vi "Full LabView Code.vi"() -> ()   [LabVIEW 2020]
uses:
  C:/Program Files (x86)/National Instruments/LabVIEW 2020/examples/Connectivity/Python/support/PythonVersionsEnum.ctl
  <vilib>/Utility/miscctls.llb/LVRectTypeDef.ctl
  <vilib>/Utility/miscctls.llb/LVPointTypeDef.ctl
  <vilib>/Instr/_visa.llb/VISA Configure Serial Port (Instr).vi
panel:
  out "final_calc":dbl
  out "Python error out":errorcluster
  in  "Python version":T1=enum."3.6"
  out "Suggested Min Electrode Separation (mm)":dbl format="%#_2g"
  out "Time for Evaporation":dbl
  out "Evaporation Rate":dbl
  out "droplet size":dbl
  out "Initial Droplet Charge":dbl
  out "Current":dbl
  in  "Flow Rate (L/min)":dbl=5e-05 min=0.0 max=1.0 step=1e-06
  in  "Voltage (V)":dbl=5000.0 min=0.0 max=5000.0 step=10.0
  in  "Solvent":enum16{"Xylene"}(ring)
  in  "Electrode separation (mm)":dbl(slide)=5.0 min=1.0 max=65.0 step=1.0
  out "Arduino Error Out":errorcluster
  out "Arduino Serial Return":string
  in  "Set":bool
  in  "Arduino COM Port":refnum<visa-resource-name>="COM5"
  in  "Stop":bool
  # "Setup"
  # "Stage Control"
  # "Spray Modelling"
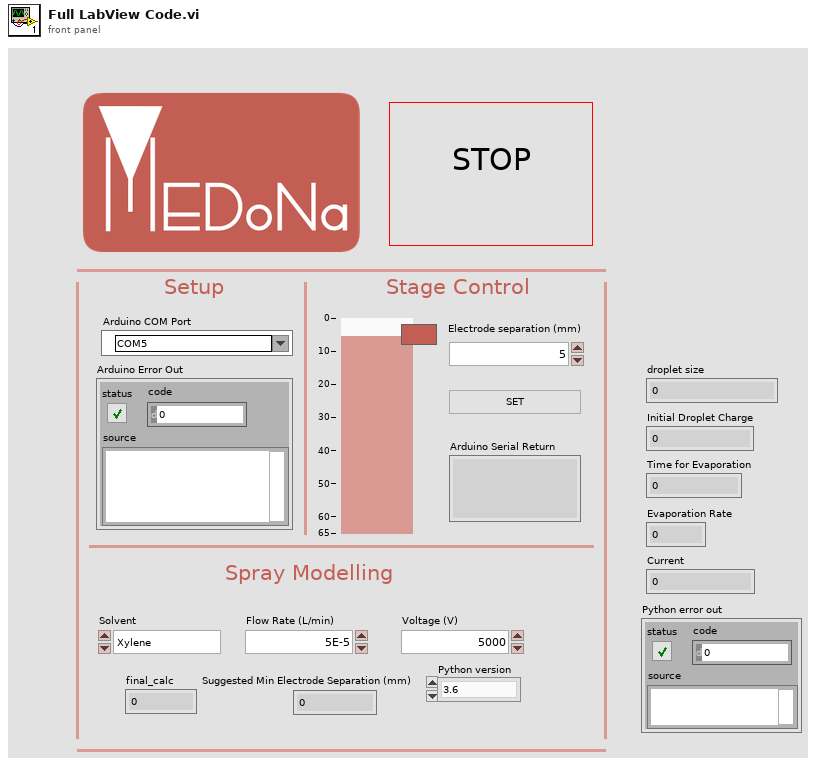
[diagram p1: front panel]
types:
  T1 = typedef "PythonVersionsEnum.ctl" = enum16{"2.7", "3.6"}
  T2 = typedef "LVRectTypeDef.ctl" = cluster{"Left":i16, "Top":i16, "Right":i16, "Bottom":i16}
  T3 = typedef "LVPointTypeDef.ctl" = cluster{"Horizontal":i16, "Vertical":i16}
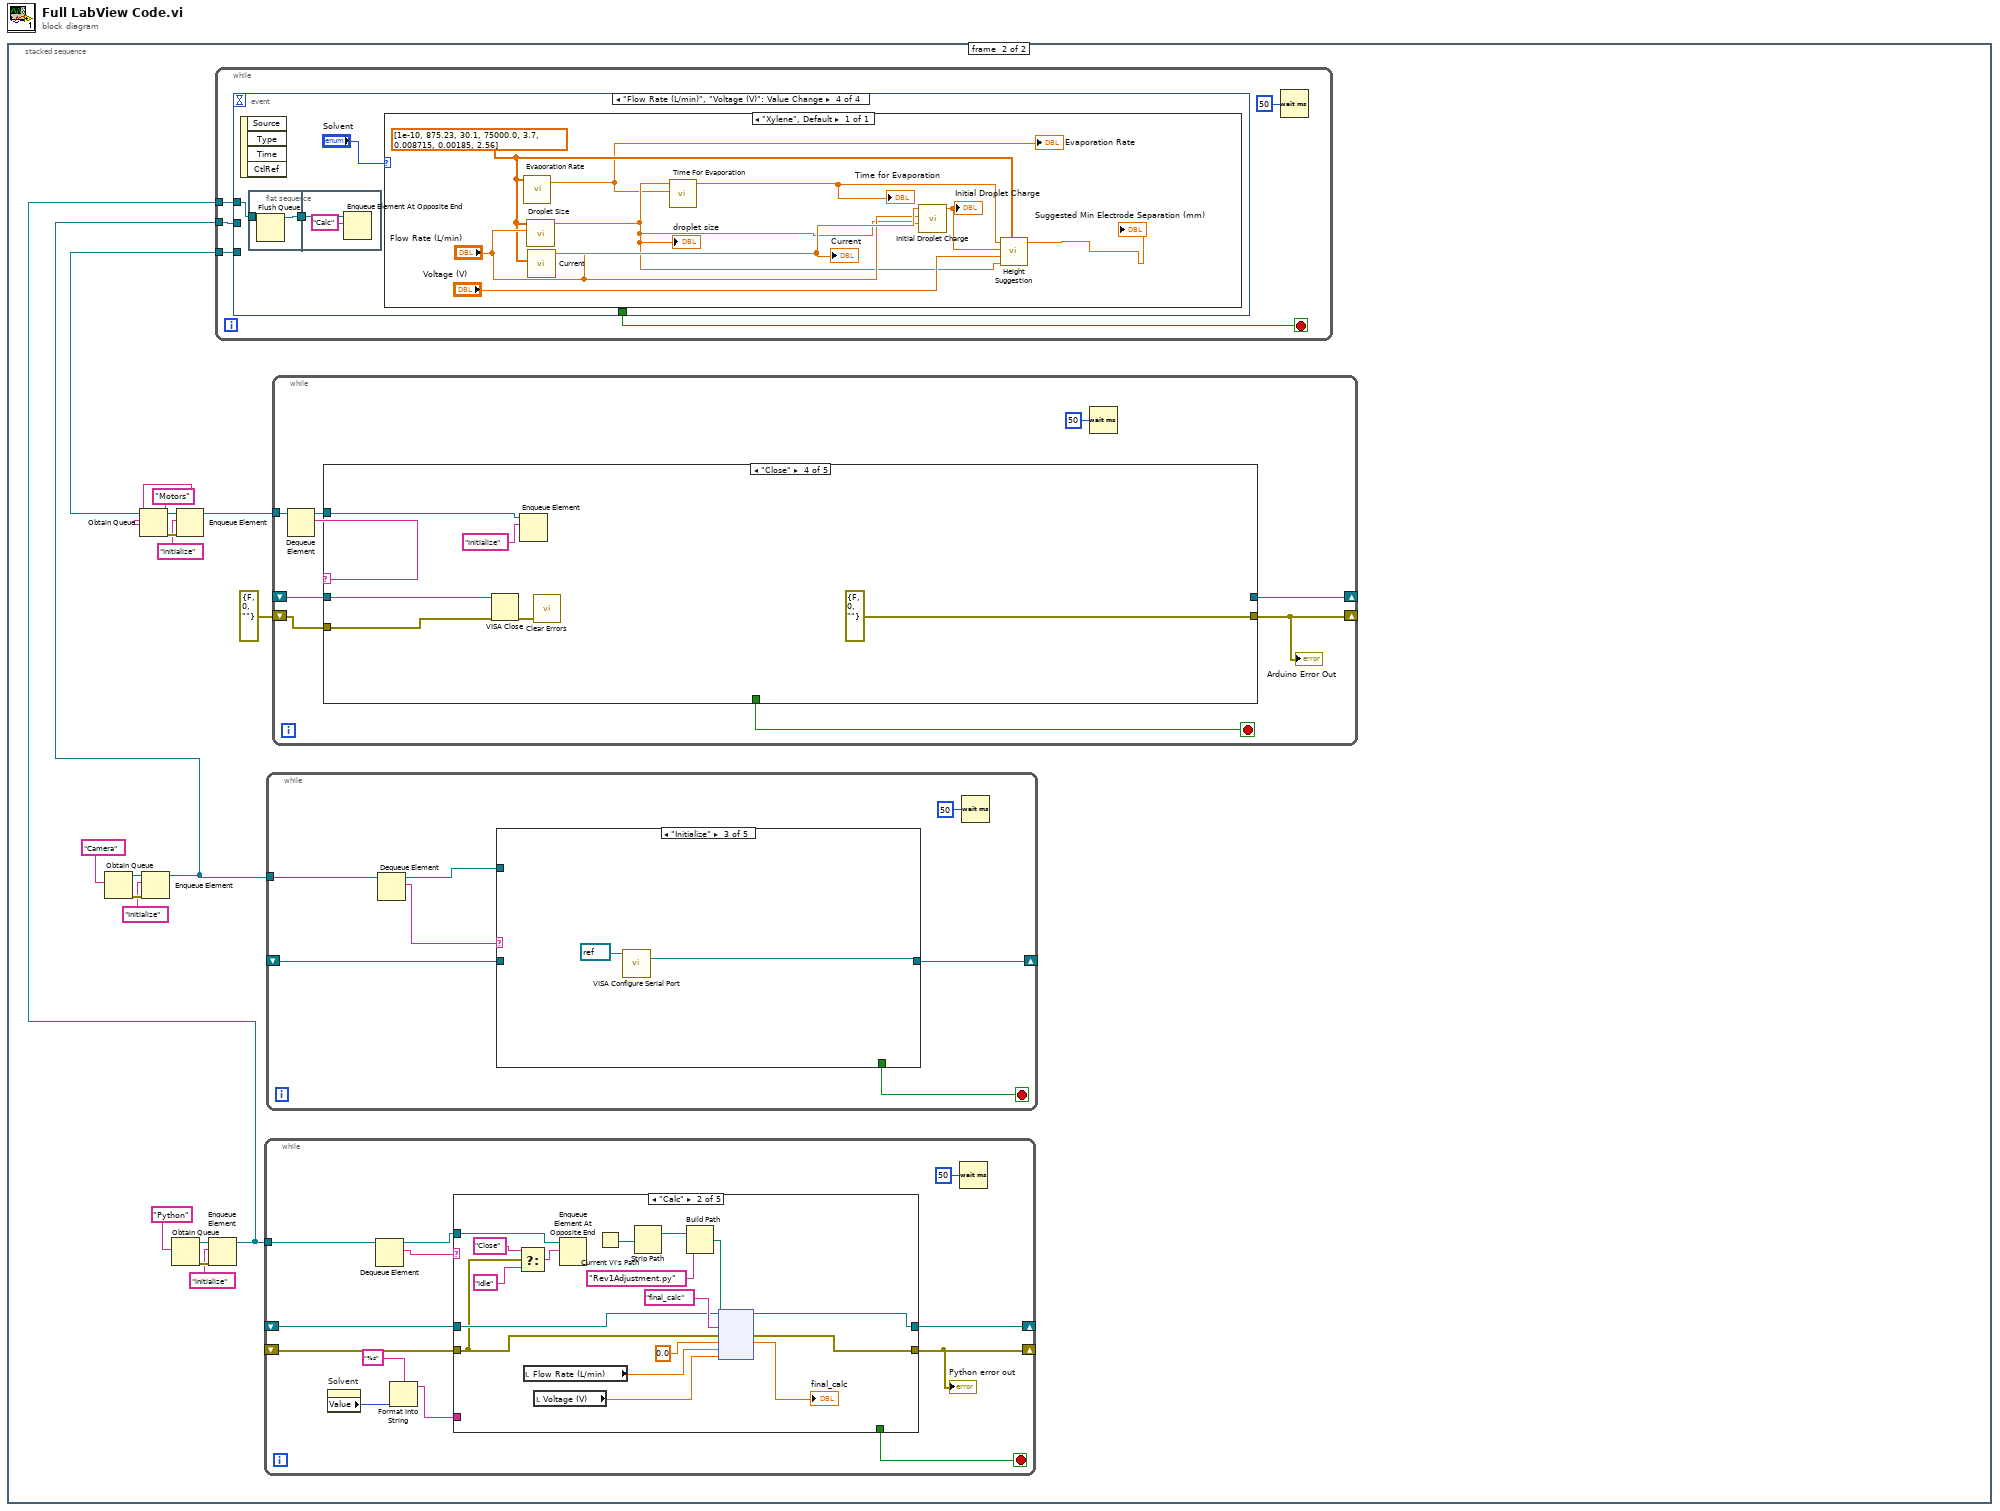
[diagram p0: block diagram]
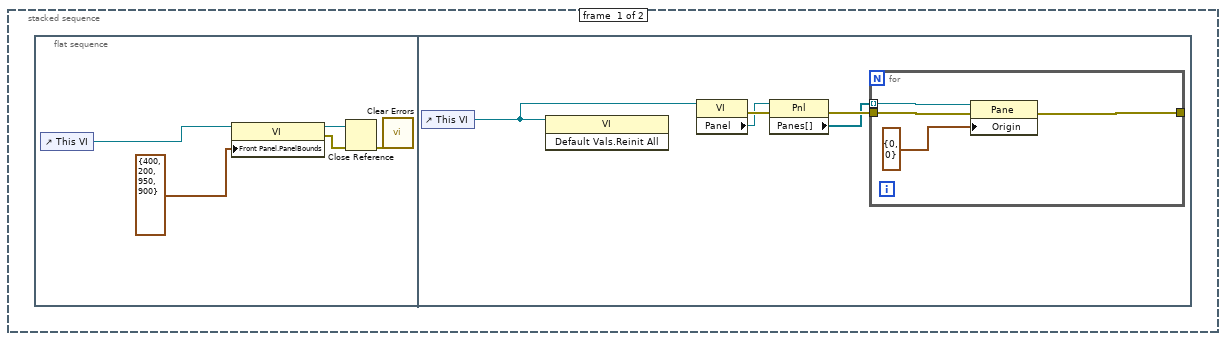
[diagram p2: hidden frame]
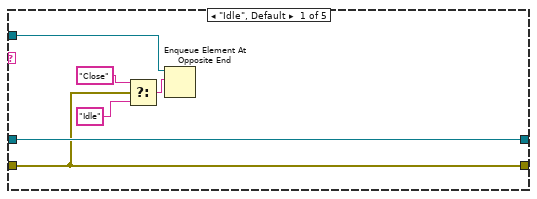
[diagram p3: hidden frame]
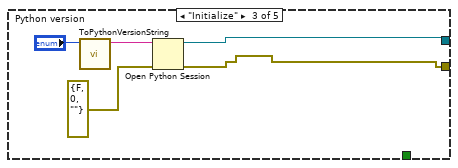
[diagram p4: hidden frame]
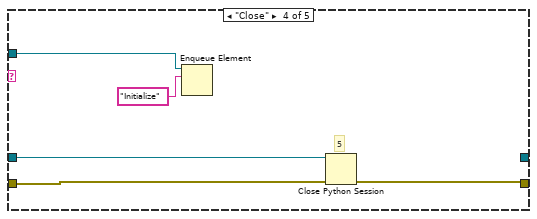
[diagram p5: hidden frame]
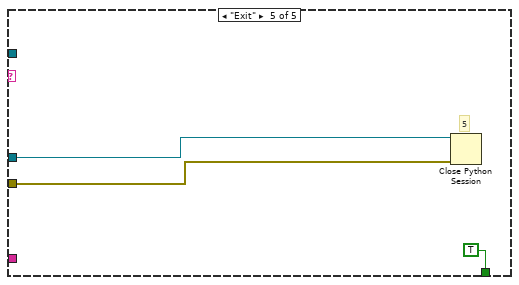
[diagram p6: hidden frame]
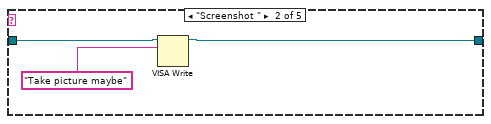
[diagram p8: hidden frame]
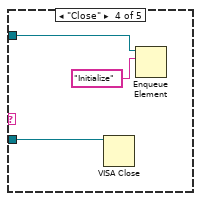
[diagram p9: hidden frame]
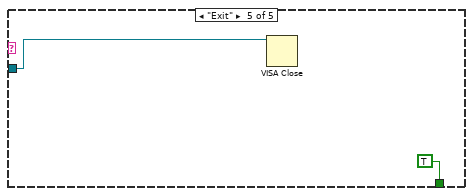
[diagram p10: hidden frame]
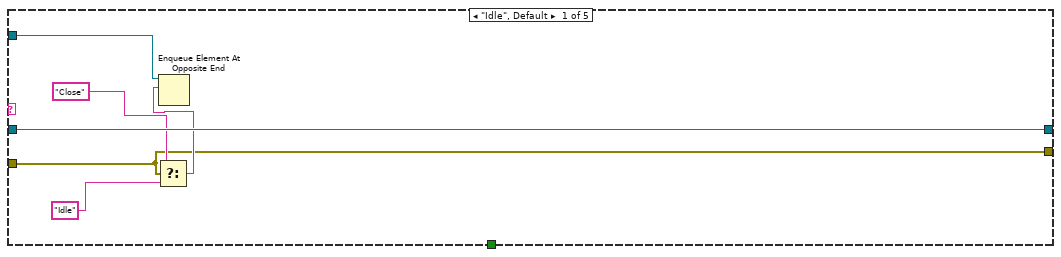
[diagram p11: hidden frame]
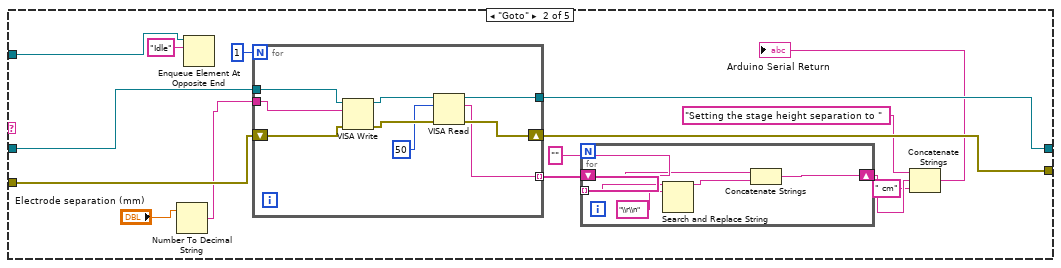
[diagram p12: hidden frame]
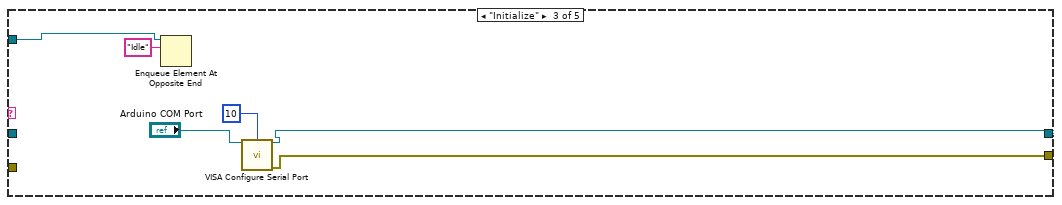
[diagram p13: hidden frame]
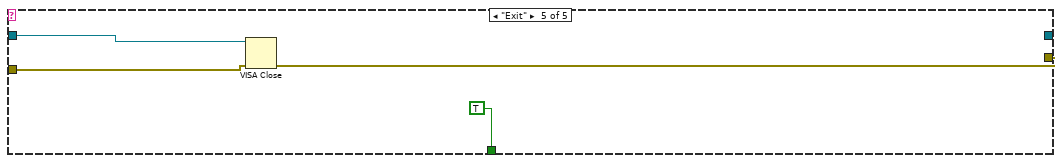
[diagram p14: hidden frame]
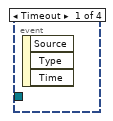
[diagram p15: hidden frame]
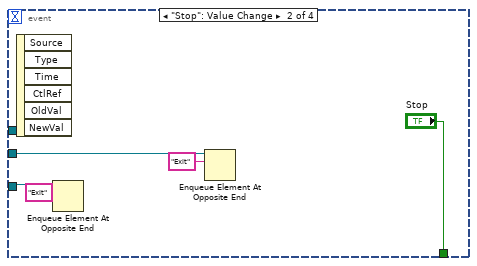
[diagram p16: hidden frame]
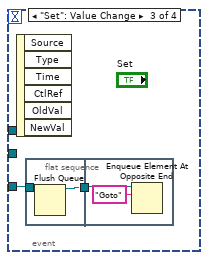
[diagram p17: hidden frame]
diagram:
  n1 = stacked-sequence {
    frame #0 {
      n2 = flat-sequence {
        frame #0 {
          n3 = control-ref of="This VI"() -> (w3:refnum<vi>)
          n4 = property class="VI"(reference=w3, "Front Panel.PanelBounds"=T2 {"Left"=400, "Top"=200, "Right"=950, "Bottom"=900} ("Front Panel Window:Panel Bounds")) -> (reference out=w5:refnum<vi>, error out=w4:errorcluster)  [unwired: 1 in]
          n5 = Close Reference(reference=w5, error in (no error)=w4) -> (error out=w1:errorcluster)
          n6 = call <vilib>:"Clear Errors.vi"("error in (no error)"=w1) -> ()  [unwired: 5 in, 2 out]
        }
        frame #1 {
          n7 = control-ref of="This VI"() -> (w10:refnum<vi>)
          n8 = invoke class="VI" method="Default Vals.Reinit All"(reference=w10) -> ()  [unwired: 2 in, 3 out]
          n9 = property class="VI"(reference=w10) -> (error out=w7:errorcluster, "Panel"=w6:refnum<vi>)  [unwired: 1 in, 1 out]
          n10 = property class="Pnl"(reference=w6, error in=w7) -> (error out=w9:errorcluster, "Panes[]"=w8:refnum<vi>[])  [unwired: 1 out]
          n11 = for {
            tunnel: w8 -> [w14] mode=indexing
            tunnel: w9 -> [w13]
            tunnel: [w11] -> _
            n12 = property class="Pane"(reference=w14, error in=w13, "Origin"=T3 {"Horizontal"=0, "Vertical"=0}) -> (error out=w11:errorcluster)  [unwired: 1 out]
          }
        }
      }
    }
    frame #1 {
      w28 = "Motors" ("name (unnamed)")
      n13 = Obtain Queue(element data type="Camera" ("name (unnamed)")) -> (queue out=w22:refnum<queue>, error out=w25:errorcluster)  [unwired: 4 in, 1 out]
      n14 = Obtain Queue(name (unnamed)=w28, element data type=w28) -> (queue out=w27:refnum<queue>, error out=w30:errorcluster)  [unwired: 3 in, 1 out]
      n15 = Enqueue Element(queue=w22, element="Initialize", error in (no error)=w25) -> (queue out=w21:refnum<queue>)  [unwired: 1 in, 2 out]
      n16 = Obtain Queue(element data type="Python" ("name (unnamed)")) -> (queue out=w16:refnum<queue>, error out=w19:errorcluster)  [unwired: 4 in, 1 out]
      n17 = Enqueue Element(queue=w27, element="Initialize", error in (no error)=w30) -> (queue out=w26:refnum<queue>)  [unwired: 1 in, 2 out]
      n18 = Enqueue Element(queue=w16, element="Initialize", error in (no error)=w19) -> (queue out=w15:refnum<queue>)  [unwired: 1 in, 2 out]
      n19 = while {
        tunnel: w27 -> [w161]
        tunnel: w21 -> [w160]
        tunnel: w15 -> [w157]
        stop <- w159 stop-if-true
        n20 = event shown="[3] \"Flow Rate (L/min)\", \"Voltage (V)\": Value Change" {
          selector: _ -> [_ _ _ _]
          dyn-events: _ -> [_ _ _ _]
          timeout: _ -> [_ _ _ _]
          tunnel: w161 -> [_ w164 w168 _]
          tunnel: w160 -> [_ w165 _ _]
          tunnel: [_ "Stop" _ _] -> w159
          tunnel: w157 -> [_ _ _ w173]
          event Timeout {
            n21 = event-data() -> ()  [unwired: 1 in, 3 out]
          }
          event "Stop": Value Change {
            n22 = event-data() -> ()  [unwired: 1 in, 6 out]
            n23 = Enqueue Element At Opposite End(queue=w164, element="Exit") -> ()  [unwired: 2 in, 3 out]
            n24 = Enqueue Element At Opposite End(queue=w165, element="Exit") -> ()  [unwired: 2 in, 3 out]
          }
          event "Set": Value Change {
            n25 = event-data() -> ()  [unwired: 1 in, 6 out]
            n26 = flat-sequence {
              tunnel: w168 -> [w170]
              tunnel: [w169] -> w167
              tunnel: w167 -> [w171]
              frame #0 {
                n27 = Flush Queue(queue=w170) -> (queue out=w169:refnum<queue>)  [unwired: 1 in, 2 out]
              }
              frame #1 {
                n28 = Enqueue Element At Opposite End(queue=w171, element="Goto") -> ()  [unwired: 2 in, 3 out]
              }
            }
          }
          event "Flow Rate (L/min)", "Voltage (V)": Value Change {
            n29 = event-data() -> ()  [unwired: 1 in, 4 out]
            n30 = flat-sequence {
              tunnel: w173 -> [w177]
              tunnel: [w176] -> w174
              tunnel: w174 -> [w178]
              frame #0 {
                n31 = Flush Queue(queue=w177) -> (queue out=w176:refnum<queue>)  [unwired: 1 in, 2 out]
              }
              frame #1 {
                n32 = Enqueue Element At Opposite End(queue=w178, element="Calc") -> ()  [unwired: 2 in, 3 out]
              }
            }
            n33 = case shown="\"Xylene\", Default" "Solvent" {
              frame "Xylene", Default {
                w182 = dbl[] [1e-10, 875.23, 30.1, 75000.0, 3.7, 0.008715, 0.00185, 2.56] ("Array 2")
                n34 = call "Evaporation Rate.vi"("array"=w182) -> ("Evaporation Rate"=w181:dbl)  [unwired: 10 in]
                "Evaporation Rate" <- w181
                n35 = call "Droplet Size.vi"("Flow Rate"="Flow Rate (L/min)", "Array"=w182) -> ("droplet size"=w183:dbl)  [unwired: 9 in]
                "droplet size" <- w183
                n36 = call "Current.vi"("array"=w182, "Flow Rate (uL/min)"="Flow Rate (L/min)") -> ("Current"=w188:dbl)  [unwired: 9 in]
                "Current" <- w188
                n37 = call "Time For Evaporation.vi"("Evaporation rate"=w181, "Droplet Size"=w183) -> ("Time for Evaporation"=w186:dbl)  [unwired: 9 in]
                "Time for Evaporation" <- w186
                n38 = call "Initial Droplet Charge.vi"("Droplet Size"=w183, "Flow Rate"="Flow Rate (L/min)", "Current"=w188) -> ("Initial Droplet Charge"=w185:dbl)  [unwired: 8 in]
                "Initial Droplet Charge" <- w185
                n39 = call "Height Suggestion.vi"("array"=w182, "Droplet Size"=w183, "Input Voltage"="Voltage (V)", "Initial Charge"=w185, "Evaporation Time"=w186) -> ("Suggested Height"=→"Suggested Min Electrode Separation (mm)":dbl)  [unwired: 6 in]
              }
            }
          }
        }
        n40 = Wait (ms)(milliseconds to wait=u32 50) -> ()  [unwired: 1 out]
      }
      n41 = while {
        tunnel: w15 -> [w42]
        shift-right: [w37] -> _
        shift-left: _ -> [w35]
        shift-right: [w34] -> _
        shift-left: _ -> [w36]
        stop <- w39 stop-if-true
        n42 = property on="Solvent" class="Enum (strict)"() -> ("Value"=w33:enum16{"Xylene"})  [unwired: 2 in, 2 out]
        n43 = Dequeue Element(queue=w42) -> (queue out=w41:refnum<queue>, element=w40:string)  [unwired: 2 in, 2 out]
        n44 = Format Into String(format string="%s", w33) -> (resulting string=w31:string)  [unwired: 2 in, 1 out]
        n45 = case shown="\"Calc\"" w40 {
          tunnel: w41 -> [w45 w49 _ w75 _]
          tunnel: [_ _ _ _ TRUE] -> w39
          tunnel: [w44 w58 w67 _ _] -> w37
          tunnel: [w43 w59 w66 w71 _] -> w34
          tunnel: w36 -> [w43 w50 _ w73 w76]
          tunnel: w35 -> [w44 w60 _ w72 w77]
          tunnel: w31 -> [_ _ _ _ _]
          frame "Idle", Default {
            n46 = Select(t="Close", s=w43, f="Idle" ("element")) -> (s? t:f=w46:string)
            n47 = Enqueue Element At Opposite End(queue=w45, element=w46) -> ()  [unwired: 2 in, 3 out]
          }
          frame "Calc" {
            n48 = Select(t="Close", s=w50, f="Idle" ("element")) -> (s? t:f=w51:string)
            n49 = local read "Flow Rate (L/min)"() -> (w57:dbl)
            n50 = local read "Voltage (V)"() -> (w56:dbl)
            n51 = Enqueue Element At Opposite End(queue=w49, element=w51) -> ()  [unwired: 2 in, 3 out]
            n52 = Current VI's Path() -> (path=w55:path)
            n53 = Strip Path(path=w55) -> (stripped path=w65:path)  [unwired: 1 out]
            n54 = Build Path(base path=w65, name or relative path="Rev1Adjustment.py") -> (appended path=w64:path)
            n55 = node(w60, w64, "final_calc" ("function name"), w50, 0.0 ("final_calc"), w57, w56) -> (w58:refnum<k35>, w59:errorcluster, →"final_calc":dbl)  [unwired: 2 in, 2 out]
          }
          frame "Initialize" {
            n56 = call "ToPythonVersionString.vi"("python version"="Python version") -> ("python version string"=w70:string)  [unwired: 10 in]
            n57 = Open Python Session(python version=w70, 3:errorcluster {"status"=FALSE, "code"=0, "source"=""} ("error in (no error)")) -> (session out=w67:refnum<k35>, error out=w66:errorcluster)  [unwired: 1 in]
          }
          frame "Close" {
            # "5"
            n58 = Enqueue Element(queue=w75, element="Initialize") -> ()  [unwired: 2 in, 3 out]
            n59 = Close Python Session(session in=w72, error in=w73) -> (11:w71:errorcluster)
          }
          frame "Exit" {
            # "5"
            n60 = Close Python Session(session in=w77, error in=w76) -> ()  [unwired: 1 out]
          }
        }
        "Python error out" <- w34
        n61 = Wait (ms)(milliseconds to wait=u32 50) -> ()  [unwired: 1 out]
      }
      n62 = while {
        tunnel: w21 -> [w85]
        shift-right: [w82] -> _
        shift-left: _ -> [w81]
        stop <- w80 stop-if-true
        n63 = Dequeue Element(queue=w85) -> (queue out=w84:refnum<queue>, element=w83:string)  [unwired: 2 in, 2 out]
        n64 = case shown="\"Initialize\"" w83 {
          tunnel: w84 -> [_ _ _ w93 _]
          tunnel: [w86 w88 w91 _ _] -> w82
          tunnel: w81 -> [w86 w89 _ w94 w96]
          tunnel: [_ _ _ _ TRUE] -> w80
          frame "Idle", Default {
            # "Run some script that Skylar has going on here"
          }
          frame "Screenshot " {
            n65 = VISA Write(VISA resource name=w89, write buffer="Take picture maybe") -> (VISA resource name out=w88:refnum<visa-resource-name>)  [unwired: 1 in, 2 out]
          }
          frame "Initialize" {
            n66 = call-poly "VISA Configure Serial Port"("VISA resource name"=refnum<visa-resource-name> refnum) -> ("VISA resource name out"=w91:refnum<visa-resource-name>)  [unwired: 13 in, 1 out]
          }
          frame "Close" {
            n67 = VISA Close(VISA resource name=w94) -> ()  [unwired: 1 in, 1 out]
            n68 = Enqueue Element(queue=w93, element="Initialize") -> ()  [unwired: 2 in, 3 out]
          }
          frame "Exit" {
            n69 = VISA Close(VISA resource name=w96) -> ()  [unwired: 1 in, 1 out]
          }
        }
        n70 = Wait (ms)(milliseconds to wait=u32 50) -> ()  [unwired: 1 out]
      }
      n71 = while {
        tunnel: w26 -> [w105]
        shift-right: [w103] -> _
        shift-left: _ -> [w102]
        shift-right: [w100] -> _
        shift-left: errorcluster {"status"=FALSE, "code"=0, "source"=""} ("error out") -> [w99]
        stop <- w101 stop-if-true
        n72 = Dequeue Element(queue=w105) -> (queue out=w98:refnum<queue>, element=w104:string)  [unwired: 2 in, 2 out]
        n73 = case shown="\"Close\"" w104 {
          tunnel: [w111 w120 w145 _ _] -> w103
          tunnel: w102 -> [w111 w124 _ w152 w156]
          tunnel: [_ _ _ _ TRUE] -> w101
          tunnel: [w106 w123 w144 errorcluster {"status"=FALSE, "code"=0, "source"=""} ("error out") w153] -> w100
          tunnel: w99 -> [w106 w122 _ w150 w154]
          tunnel: w98 -> [w107 w115 w142 w148 _]
          frame "Idle", Default {
            n74 = Select(t="Close" ("element"), s=w106, f="Idle" ("element")) -> (s? t:f=w108:string)
            n75 = Enqueue Element At Opposite End(queue=w107, element=w108) -> ()  [unwired: 2 in, 3 out]
          }
          frame "Goto" {
            n76 = Number To Decimal String(number="Electrode separation (mm)") -> (decimal integer string=w113:string)  [unwired: 1 in]
            n77 = Enqueue Element At Opposite End(queue=w115, element="Idle") -> ()  [unwired: 2 in, 3 out]
            n78 = for {
              N: 1 -> [_]
              shift-right: [w137] -> w123
              shift-left: w122 -> [w139]
              tunnel: [w136] -> w126 mode=indexing
              tunnel: w124 -> [w135]
              tunnel: [w134] -> w120
              tunnel: w113 -> [w132]
              n79 = VISA Write(VISA resource name=w135, write buffer=w132, error in (no error)=w139) -> (VISA resource name out=w140:refnum<visa-resource-name>, error out=w138:errorcluster)  [unwired: 1 out]
              n80 = VISA Read(VISA resource name=w140, byte count=u32 50, error in (no error)=w138) -> (VISA resource name out=w134:refnum<visa-resource-name>, read buffer=w136:string, error out=w137:errorcluster)  [unwired: 1 out]
            }
            n81 = for {
              tunnel: w126 -> [w127] mode=indexing
              shift-right: [w131] -> w118
              shift-left: "" -> [w130]
              n82 = Search and Replace String(input string=w127, search string="\\r\\n") -> (result string=w128:string)  [unwired: 6 in, 3 out]
              n83 = Concatenate Strings(w130, w128) -> (w131:string)
            }
            n84 = Concatenate Strings("Setting the stage height separation to " ("string"), w118, " cm" ("string")) -> (→"Arduino Serial Return":string)
          }
          frame "Initialize" {
            n85 = Enqueue Element At Opposite End(queue=w142, element="Idle") -> ()  [unwired: 2 in, 3 out]
            n86 = call-poly "VISA Configure Serial Port"("VISA resource name"="Arduino COM Port", "termination char\n(0xA = '\\n' = LF)"=u8 10 ("termination char\n(0xA = '\\n' = LF)")) -> ("VISA resource name out"=w145:refnum<visa-resource-name>, "error out"=w144:errorcluster)  [unwired: 12 in]
          }
          frame "Close" {
            n87 = VISA Close(VISA resource name=w152, error in (no error)=w150) -> (error out=w147:errorcluster)
            n88 = Enqueue Element(queue=w148, element="Initialize") -> ()  [unwired: 2 in, 3 out]
            n89 = call <vilib>:"Clear Errors.vi"("error in (no error)"=w147) -> ()  [unwired: 5 in, 2 out]
          }
          frame "Exit" {
            n90 = VISA Close(VISA resource name=w156, error in (no error)=w154) -> (error out=w153:errorcluster)
          }
        }
        "Arduino Error Out" <- w100
        n91 = Wait (ms)(milliseconds to wait=u32 50) -> ()  [unwired: 1 out]
      }
    }
  }
